vi "zi_S1_S2.vi"(0 "Address":string="DEV1925", 1 "stop":bool) -> ()   [LabVIEW 2021]
doc: "Control a Zurich instrument device via the LabOne Labview API. \nRequirements: Zurich Instruments MFLI, HF2 or UHFLI \nThis example polls demod data for a given time from the instrument.\n\n© Zurich Instruments AG, www.zhinst.com"
uses:
  <vilib>/Analysis/1siggen.llb/Ramp Pattern by Samples.vi
  <instrlib>/Zurich Instruments LabOne/Public/Configure/ziSetValueDouble.vi
  <instrlib>/Zurich Instruments LabOne/Public/Configure/ziGetValueDouble.vi
  <instrlib>/Zurich Instruments LabOne/Public/Utility/ziTicksToS_vector.vi
  <instrlib>/Zurich Instruments LabOne/Zurich Instruments LabOne.lvlib
  <vilib>/Analysis/NI_AALBase.lvlib
panel:
  in  "Update V":bool
  out "Current V":dbl=0.24999427791044548
  in  "N samples":dbl=10.0
  out "Waveform Chart":dbl[][](graph)
  in  "Ending V":dbl=0.25
  in  "Starting V":dbl=0.2
  out "Error Out":errorcluster
  out "XY Graph":cluster{dbl[], "X (Vrms)":dbl[]}[](graph)
  in  "time":dbl=3.0 caption="recording time [s]"
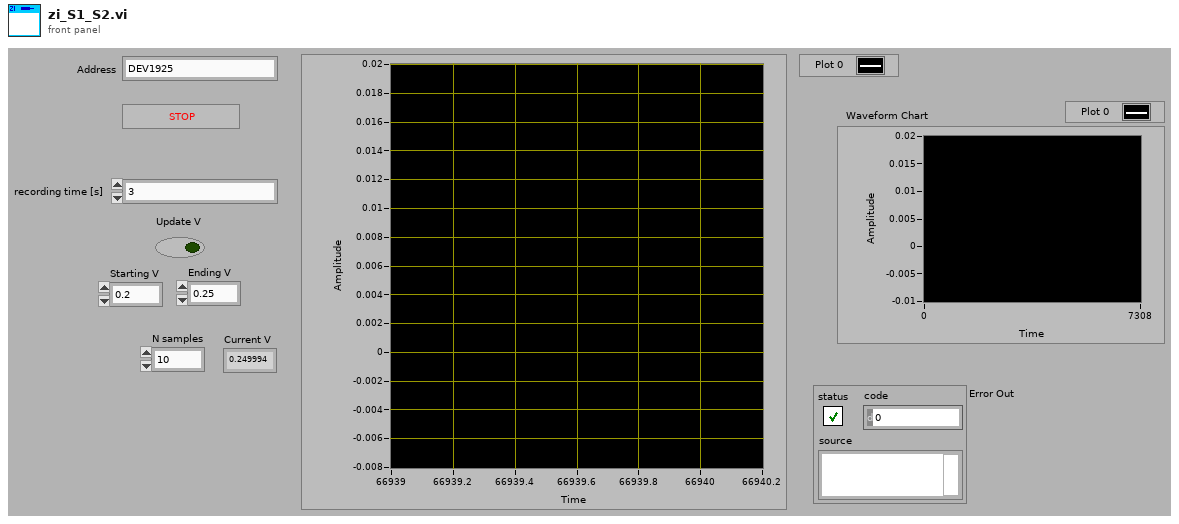
[diagram p1: front panel]
types:
  T1 = typedef "Zurich Instruments LabOne.lvlib/ziTypeHandle.ctl" = cluster{"handleValid":bool, "Conn":u64, "Path Prefix":string, "Handle":u64, "Connected":bool, "Clockbase(s)":dbl}
  T2 = typedef "Zurich Instruments LabOne.lvlib/ziTypeDemodSampleEx.ctl" = cluster{"Timestamps (ticks)":u64[], "X (Vrms)":dbl[], "Y (Vrms)":dbl[], "Osc Phase (rad)":dbl[], "Freq (Hz)":dbl[], "DIO":u32[], "Aux In 0 (V)":dbl[], "Aux In 1 (V)":dbl[], "Trigger":u32[]}
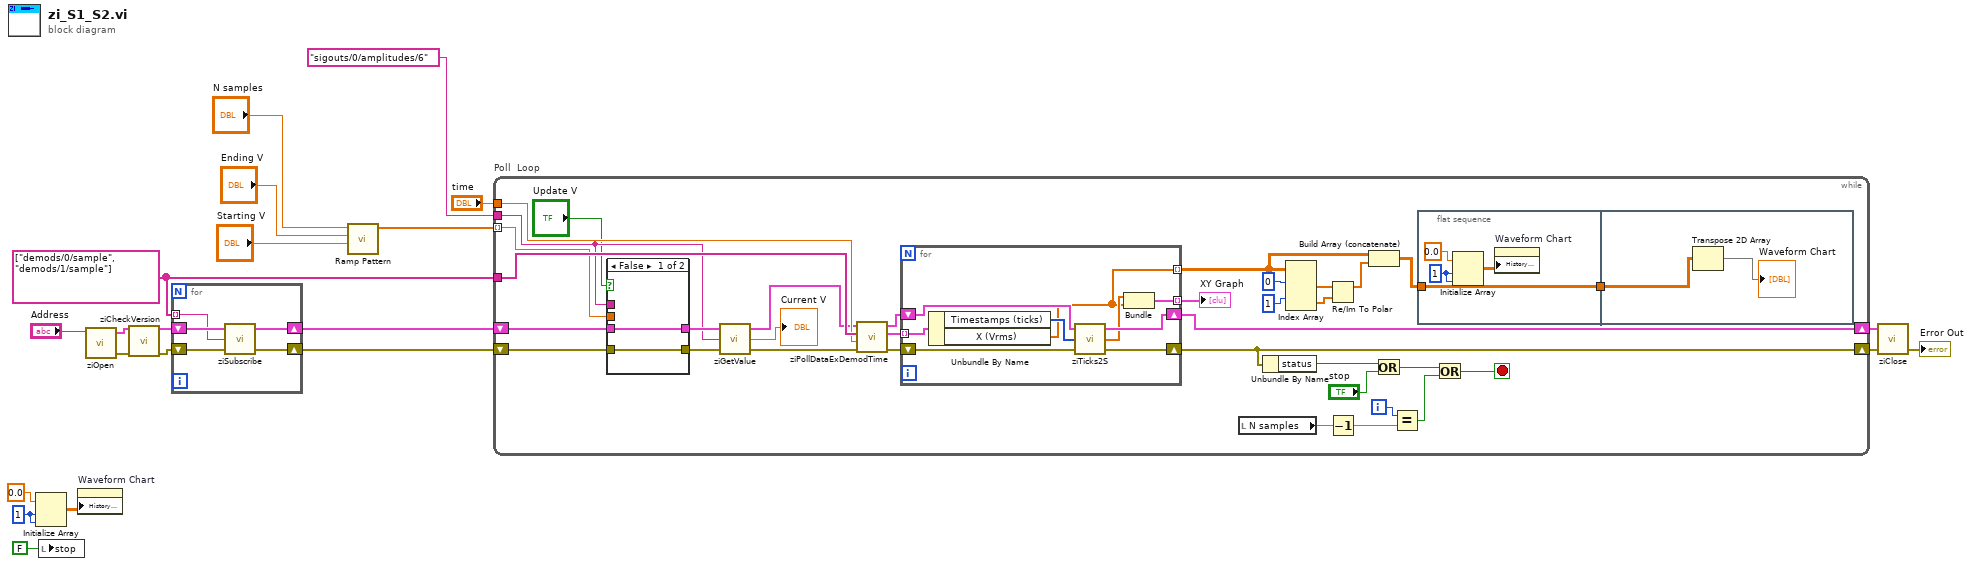
[diagram p0: block diagram]
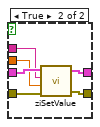
[diagram p2: hidden frame]
diagram:
  w1 = 1
  w9 = string[] ["demods/0/sample", "demods/1/sample"]
  n1 = Initialize Array(0.0, w1, w1) -> (w2:dbl[][])
  n2 = local write "stop"(FALSE ("stop")) -> ()
  n3 = property on="Waveform Chart" class="WFChart (strict)"("History Data"=w2) -> ()  [unwired: 2 in, 2 out]
  n4 = call <instrlib>:"ziOpen.vi"("Address"="Address") -> ("Error Out"=w12:errorcluster, "HandleOut"=w13:T1)  [unwired: 1 in, 3 out]
  n5 = call <instrlib>:"ziCheckVersion.vi"("Handle In"=w13, "Error In"=w12) -> ("Handle Out"=w10:T1, "Error Out"=w11:errorcluster)  [unwired: 11 in, 1 out]
  n6 = for {
    tunnel: w9 -> [w22] mode=indexing
    shift-right: [w24] -> w17
    shift-left: w11 -> [w25]
    shift-right: [w23] -> w16
    shift-left: w10 -> [w26]
    n7 = call <instrlib>:"ziSubscribe.vi"("error in"=w25, "Path ()"=w22, "Handle In"=w26) -> ("error out"=w24:errorcluster, "Handle Out"=w23:T1)  [unwired: 1 in]
  }
  n8 = call-poly <vilib>:"Ramp Pattern.vi"("start"="Starting V", "end"="Ending V", "samples"="N samples") -> ("Ramp Pattern"=w4:dbl[])  [unwired: 7 in, 1 out]
  n9 = while "Poll  Loop" {
    shift-right: [w57] -> w21
    shift-left: w16 -> [w51]
    shift-right: [w53] -> w19
    shift-left: w17 -> [w50]
    tunnel: w9 -> [w60]
    tunnel: "time" -> [w55]
    tunnel: "sigouts/0/amplitudes/6" -> [w39]
    tunnel: w4 -> [w44] mode=indexing
    i -> [w45]
    stop <- w48 stop-if-true
    n10 = case shown="False" "Update V" {
      tunnel: w51 -> [w62 w68]
      tunnel: w50 -> [w61 w67]
      tunnel: w44 -> [_ w66]
      tunnel: [w62 w65] -> w40
      tunnel: w39 -> [_ w64]
      tunnel: [w61 w63] -> w37
      frame False {
      }
      frame True {
        n11 = call-poly <instrlib>:"ziSetValue.vi"("Error In"=w67, "Value"=w66, "Path"=w64, "Handle In"=w68) -> ("Error Out"=w63:errorcluster, "Handle Out"=w65:T1)  [unwired: 1 in]
      }
    }
    n12 = call-poly <instrlib>:"ziGetValue.vi"("error in"=w37, "Path"=w39, "Handle in"=w40) -> ("error out"=w36:errorcluster, "Value"=→"Current V":dbl, "Handle out"=w38:T1)
    n13 = call <instrlib>:"ziPollDataExDemodTime.vi"("error in"=w36, "recording time (1) [s]"=w55, "SubscribepathArray"=w60, "Handle In"=w38) -> ("error out"=w59:errorcluster, "Demod Sample Out"=w56:T2[], "Handle Out"=w58:T1)  [unwired: 5 in]
    n14 = for {
      tunnel: w56 -> [w79] mode=indexing
      shift-right: [w80] -> w53
      shift-left: w59 -> [w83]
      shift-right: [w81] -> w57
      shift-left: w58 -> [w82]
      tunnel: [w77] -> w54 mode=indexing
      tunnel: [w75] -> w29 mode=indexing
      n15 = Unbundle By Name(w79) -> ("Timestamps (ticks)"=w78:u64[], "X (Vrms)"=w75:dbl[])
      n16 = call-poly <instrlib>:"ziTicks2S.vi"("Error In"=w83, "Timestamp (ticks)"=w78, "Handle In"=w82) -> ("Error Out"=w80:errorcluster, "Timestamp(s)"=w76:dbl[], "Handle Out"=w81:T1)
      n17 = Bundle("Timestamp(s)"=w76, "X (Vrms)"=w75) -> (w77:cluster{"Timestamp(s)":dbl[], "X (Vrms)":dbl[]})  [unwired: 1 in]
    }
    "XY Graph" <- w54
    n18 = local read "N samples"() -> (w43:dbl)
    n19 = Unbundle By Name(w53) -> ("status"=w52:bool)
    n20 = Index Array(array=w29, index (row) #1=0, index (row) #2=1) -> (element #1=w31:dbl[], element #2=w30:dbl[])  [unwired: 2 in]
    n21 = Re/Im To Polar(2:w30, 3:w31) -> (1:w28:dbl[])  [unwired: 1 out]
    n22 = Decrement(x=w43) -> (x-1=w42:dbl)
    n23 = Build Array (concatenate)(w29, w28) -> (w27:dbl[][])
    n24 = Or(x=w52, y="stop") -> (x .or. y?=w49:bool)
    n25 = Equal?(x=w45, y=w42) -> (x = y?=w46:bool)
    n26 = flat-sequence {
      tunnel: w27 -> [w72]
      tunnel: [w72] -> w33
      tunnel: w33 -> [w74]
      frame #0 {
        w69 = 1
        n27 = Initialize Array(0.0, w69, w69) -> (w71:dbl[][])
        n28 = property on="Waveform Chart" class="WFChart (strict)"("History Data"=w71) -> ()  [unwired: 2 in, 2 out]
      }
      frame #1 {
        n29 = Transpose 2D Array(2D array=w74) -> (transposed array=→"Waveform Chart":dbl[][])
      }
    }
    n30 = Or(x=w49, y=w46) -> (x .or. y?=w48:bool)
  }
  n31 = call <instrlib>:"ziClose.vi"("Error In"=w19, "Handle In"=w21) -> ("Error Out"=→"Error Out":errorcluster)  [unwired: 3 out]
